vi "Percentual error FFT.vi"(8 "Detected Freq":dbl, 9 "#Periods":dbl=100.0, 10 "Gen. Freq.":dbl=10000000.0 format="%#_13g", 11 "#Samples":dbl=1024.0) -> (1 "Error %":dbl, 2 "Theoretical Freq.":dbl)   [LabVIEW 2014]
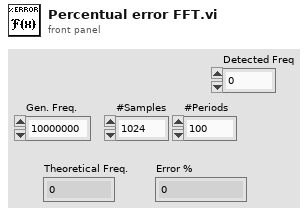
[diagram p1: front panel]
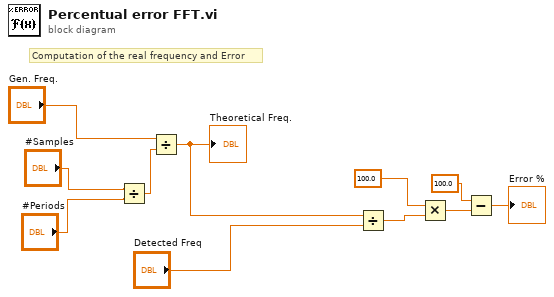
[diagram p0: block diagram]
diagram:
  # "Computation of the real frequency and Error"
  n1 = Divide(x="#Samples", y="#Periods") -> (x/y=w11:dbl)
  n2 = Divide(x="Gen. Freq.", y=w11) -> (x/y=w10:dbl)
  "Theoretical Freq." <- w10
  n3 = Divide(x=w10, y="Detected Freq") -> (x/y=w9:dbl)
  n4 = Multiply(x=100.0, y=w9) -> (x*y=w5:dbl)
  n5 = Subtract(x=100.0, y=w5) -> (x-y=→"Error %":dbl)
